vi "Digitizer Scan Fetch Period.vi"(6 "Channel":string, 7 "LastPoint":i32 format="%.0g", 8 "error in (no error)":errorcluster {"code" format="%.0x"}, 9 "FirstPoint":i32 format="%.0g", 10 "Record":i32 format="%.0g", 11 "instrument handle":refnum<k15>) -> (0 "error out":errorcluster {"code" format="%.0x"}, 2 "Val":dbl, 3 "instrument handle out":refnum<k15>)   [LabVIEW 2020, in "Keysight DAQ970.lvlib"]
doc: "Performs post-processing calculation on the specified range of readings and returns period on the specified record for a channel."
uses:
  Keysight DAQ970.lvlib
  KtDAQ970.dll
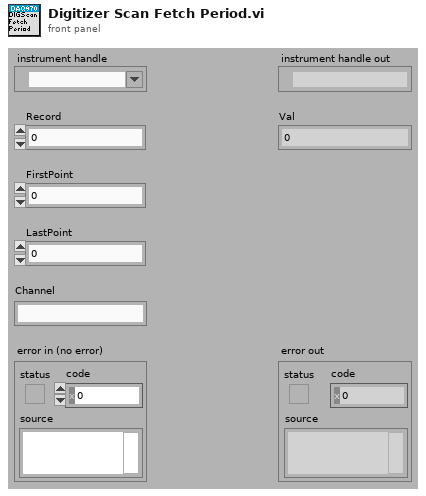
[diagram p1: front panel]
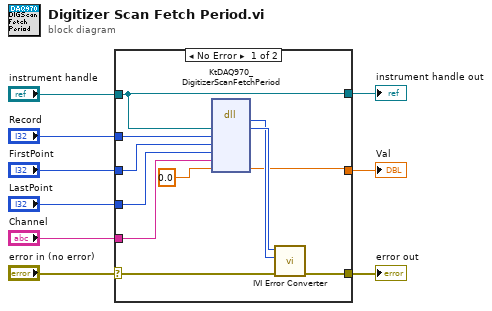
[diagram p0: block diagram]
diagram:
  n1 = case shown="No Error" "error in (no error)" {
    selector: "error in (no error)" -> [w18 w22]
    tunnel: [w17 w22] -> w9
    tunnel: "instrument handle" -> [w10 w21]
    tunnel: "Record" -> [w16 _]
    tunnel: "FirstPoint" -> [w15 _]
    tunnel: "LastPoint" -> [w14 _]
    tunnel: "Channel" -> [w13 _]
    tunnel: [w11 _] -> w2
    tunnel: [w10 w21] -> w1
    frame No Error {
      n2 = dll-call lib="KtDAQ970**.dll" fn="KtDAQ970_DigitizerScanFetchPeriod"("Vi"=w10, "Record"=w16, "FirstPoint"=w15, "LastPoint"=w14, "Channel"=w13, "Val"=0.0) -> (w19:i32, "Vi"=w20:u32, "Val"=w11:dbl)  [unwired: 7 in, 2 out]
      n3 = call "IVI Error Converter.vi"("error in (no error)"=w18, "IVI error code (0)"=w19, "instrument handle"=w20) -> ("error out"=w17:errorcluster)  [unwired: 7 in, 1 out]
    }
    frame Error {
    }
  }
  "error out" <- w9
  "instrument handle out" <- w1
  "Val" <- w2
